vi "FS-Packet over Ethernet Duplex.vi"() -> ()   [LabVIEW 2018]
uses:
  FGV Mode.ctl
  <vilib>/Utility/error.llb/DialogType.ctl
  <instrlib>/niUSRP/niUSRP Write Tx Data (I16).vi
  <instrlib>/niUSRP/niUSRP Fetch Rx Data (I16).vi
panel:
  in  "タブ制御器":enum32{"Settings", "Readback"}(tab)
  in  "device names":refnum<k15>="192.168.1.51"
  in  "number of samples":i64=2000
  in  "IQ rate":dbl=100000.0 format="%#_6p"
  in  "rx carrier frequency":dbl=2000000000.0 format="%#_6p"
  in  "rx gain":dbl format="%#_6f"
  in  "tx gain":dbl format="%#_6f"
  in  "tx carrier frequency":dbl=2000000000.0 format="%#_6p"
  in  "dstaddr":string="192.168.0.112" caption="IQデータ送信先のIPアドレス"
  in  "dsrport":i32=40000 caption="IQデータ送信先のポート番号"
  in  "srcaddr":string="192.168.0.109" caption="IQデータを受信するIPアドレス"
  in  "srcport":i32=40000 caption="IQデータを受信するポート番号"
  in  "UDP socket buffer size (recv)":i32=64000
  in  "rx buff size (max)":i32=500 caption="USRP受信用バッファサイズ"
  in  "USRP送信用バッファサイズ":i32=500
  out "rx buffer (current)":i32
  out "tx buffer (current)":i32
  out "UDP recv bytes":i32
  out "rx IQ rate":dbl=100000.0 format="%#_6p"
  out "rx carrier frequency":dbl=2000000000.0 format="%#_6p"
  out "rx gain 2":dbl format="%#_6f"
  out "tx IQ rate":dbl=100000.0 format="%#_6p"
  out "tx carrier frequency":dbl=2000000000.0 format="%#_6p"
  out "tx gain 2":dbl format="%#_6f"
  out "udp tx loop":errorcluster
  out "udp rx loop":errorcluster
  out "usrp tx loop":errorcluster
  out "usrp rx loop":errorcluster
  in  "停止":bool
  out "UDP Recv timeout":bool
  out "tx buffer full":bool caption="tx buffer full (UDP - USRP)"
  out "rx buffer full":bool caption="rx buffer full (USRP - UDP)"
  out "IQ data":i16[](array[numeric])
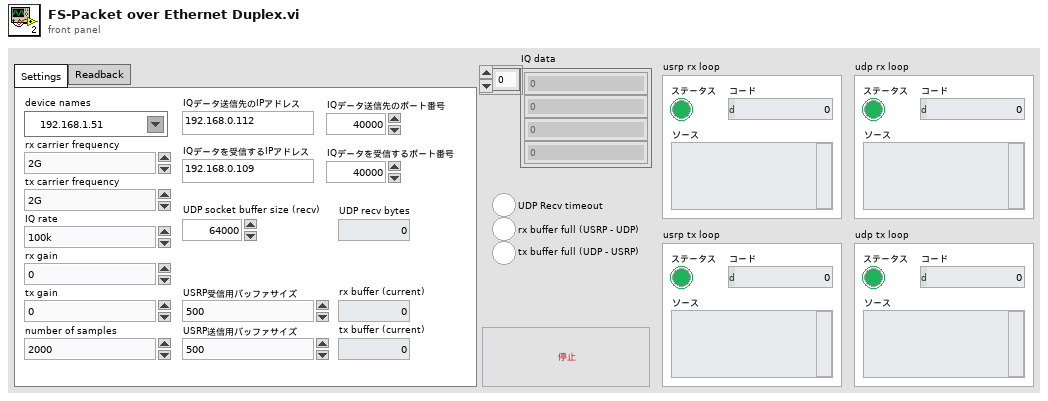
[diagram p1: front panel]
types:
  T1 = typedef "FGV Mode.ctl" = enum16{"None", "Init", "Set", "Get", "Update", "Clear"}
  T2 = typedef "DialogType.ctl" = u16
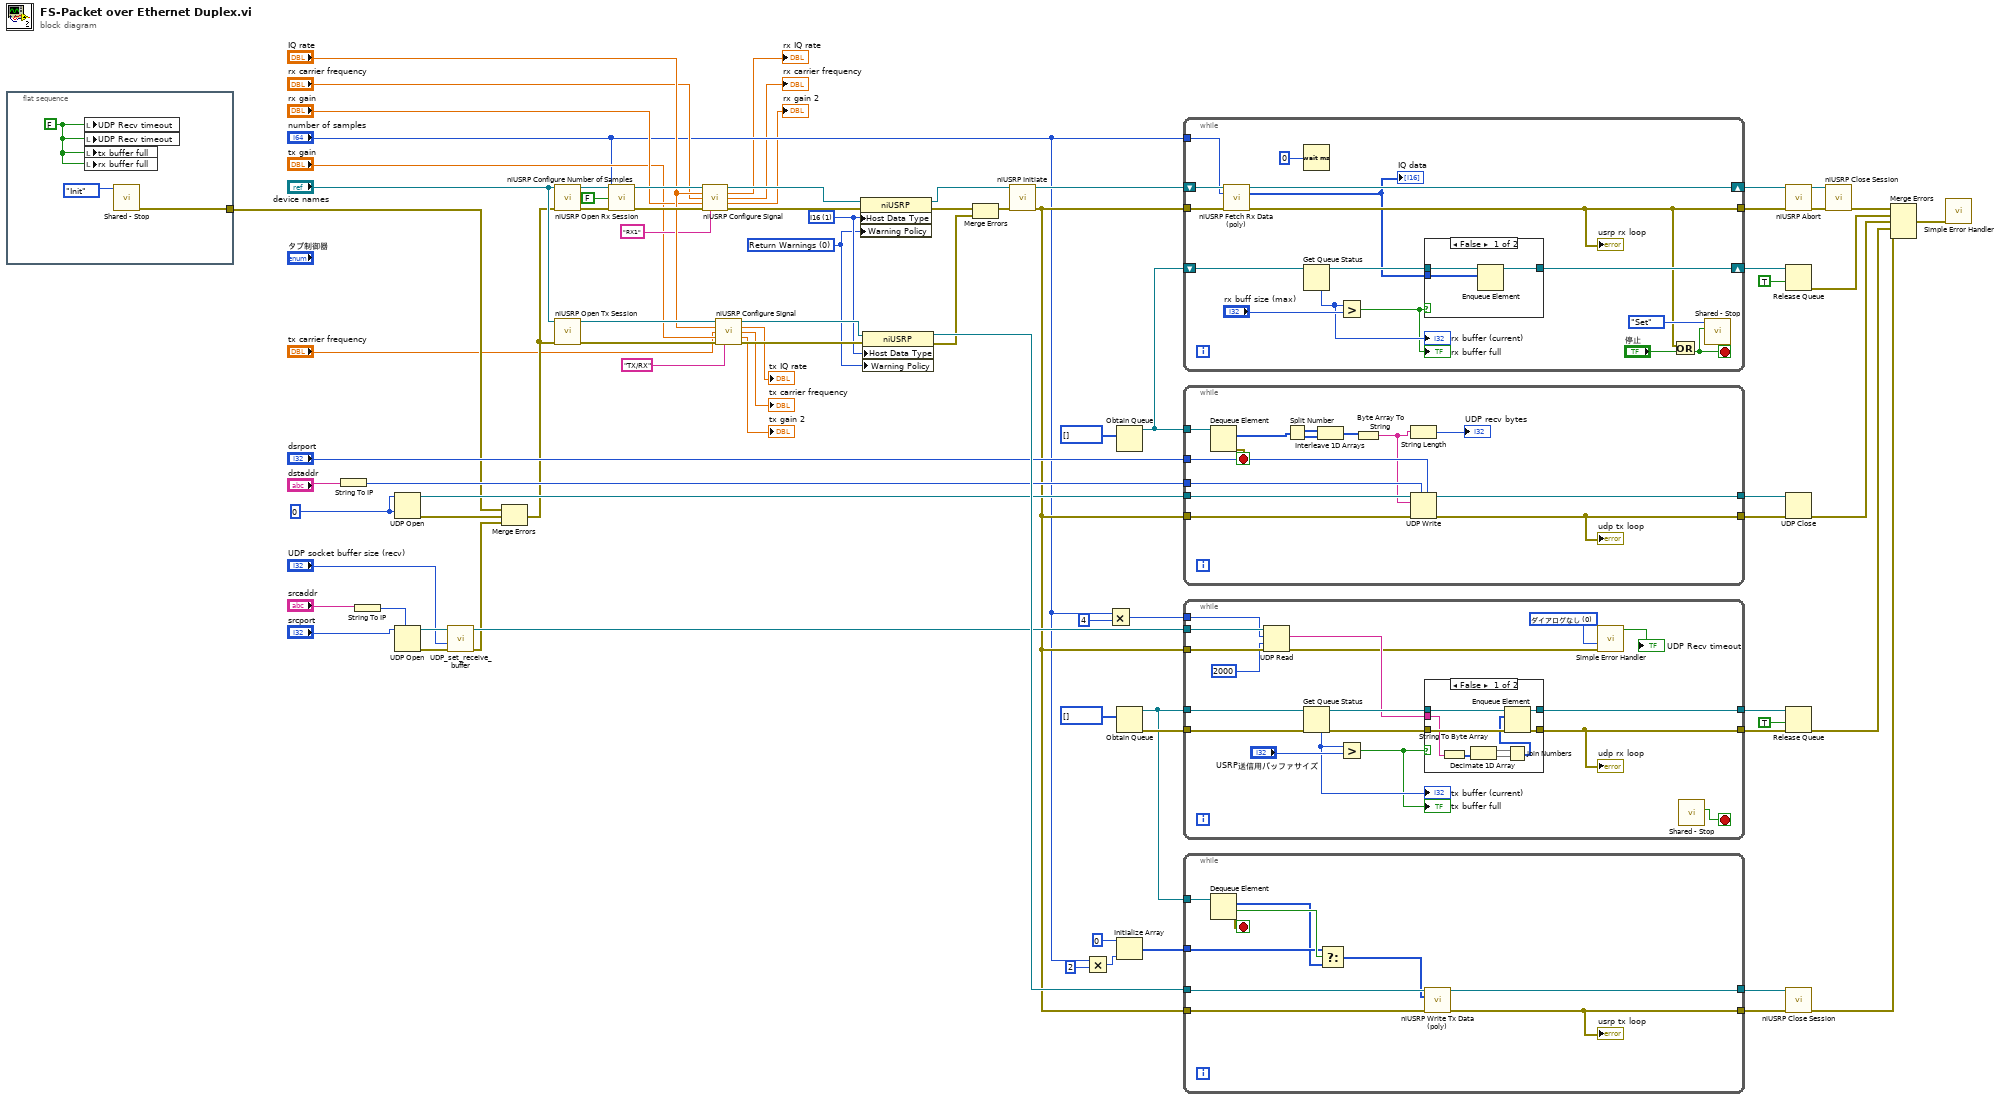
[diagram p0: block diagram]
diagram:
  w47 = u32 0 ("ネットアドレス")
  w18 = 0 items=["Return Warnings", "Return Errors", "Return Success"] ("Configuration:Advanced:Warning Policy")
  w19 = 1 items=["CDB", "I16"] ("Configuration:Advanced:Host Data Type")
  n1 = flat-sequence {
    tunnel: [w82] -> w25
    frame #0 {
      w84 = FALSE ("USRP rx overflow")
      n2 = local write "UDP Recv timeout"(w84) -> ()
      n3 = local write "UDP Recv timeout"(w84) -> ()
      n4 = local write "tx buffer full"(w84) -> ()
      n5 = local write "rx buffer full"(w84) -> ()
      n6 = call "Shared - Stop.vi"("FGV Mode"=FGV_Mode."Init") -> ("error out"=w82:errorcluster)  [unwired: 9 in, 1 out]
    }
  }
  n7 = String To IP(1:"dstaddr") -> (0:w49:u32)
  n8 = String To IP(1:"srcaddr") -> (0:w43:u32)
  n9 = UDP Open(7:w47, 11:w47) -> (port=w52:refnum<k16>, 0:w31:errorcluster)  [unwired: 3 in, 1 out]
  n10 = UDP Open(7:w43, 11:"srcport") -> (port=w36:refnum<k16>, 0:w35:errorcluster)  [unwired: 3 in, 1 out]
  n11 = call "UDP_set_receive_buffer.vi"("error in (no error)"=w35, "Receive Buffer Size"="UDP socket buffer size (recv)", "connection ID"=w36) -> ("error out"=w24:errorcluster, "connection ID out"=w34:refnum<k16>)  [unwired: 6 in]
  n12 = Merge Errors(w25, w31, w24) -> (w23:errorcluster)
  n13 = call <instrlib>:"niUSRP Open Rx Session.vi"("device names"="device names", "error in (no error)"=w23) -> ("session handle out"=w81:refnum<k15>, "error out"=w72:errorcluster)  [unwired: 12 in]
  n14 = call <instrlib>:"niUSRP Open Tx Session.vi"("device names"="device names", "error in (no error)"=w23) -> ("session handle out"=w69:refnum<k15>, "error out"=w68:errorcluster)  [unwired: 12 in]
  n15 = call <instrlib>:"niUSRP Configure Number of Samples.vi"("session handle"=w81, "number of samples is finite"=FALSE, "number of samples"="number of samples", "error in (no error)"=w72) -> ("session handle out"=w80:refnum<k15>, "error out"=w73:errorcluster)  [unwired: 10 in]
  n16 = call <instrlib>:"niUSRP Configure Signal.vi"("session handle"=w80, "IQ rate"="IQ rate", "carrier frequency"="rx carrier frequency", "gain"="rx gain", "error in (no error)"=w73, "active antenna"="RX1") -> ("session handle out"=w79:refnum<k15>, "coerced IQ rate"=→"rx IQ rate":dbl, "coerced carrier frequency"=→"rx carrier frequency":dbl, "coerced gain"=→"rx gain 2":dbl, "error out"=w59:errorcluster)  [unwired: 5 in]
  n17 = call <instrlib>:"niUSRP Configure Signal.vi"("session handle"=w69, "IQ rate"="IQ rate", "carrier frequency"="tx carrier frequency", "gain"="tx gain", "error in (no error)"=w68, "active antenna"="TX/RX") -> ("session handle out"=w58:refnum<k15>, "coerced IQ rate"=→"tx IQ rate":dbl, "coerced carrier frequency"=→"tx carrier frequency":dbl, "coerced gain"=→"tx gain 2":dbl, "error out"=w56:errorcluster)  [unwired: 5 in]
  n18 = property class="niUSRP"(reference=w79, error in=w59, "Host Data Type"=w19, "Warning Policy"=w18) -> (reference out=w60:refnum<k15>, error out=w30:errorcluster)
  n19 = property class="niUSRP"(reference=w58, error in=w56, "Host Data Type"=w19, "Warning Policy"=w18) -> (reference out=w57:refnum<k15>, error out=w21:errorcluster)
  n20 = Merge Errors(w30, w21) -> (w22:errorcluster)
  n21 = call <instrlib>:"niUSRP Initiate.vi"("session handle"=w60, "error in (no error)"=w22) -> ("session handle out"=w78:refnum<k15>, "error out"=w20:errorcluster)  [unwired: 12 in]
  n22 = Multiply(x="number of samples", y=i16 2) -> (x*y=w9:i64)
  n23 = Multiply(x="number of samples", y=4 ("最大サイズ (548)")) -> (x*y=w28:i64)
  n24 = Obtain Queue(element data type=i16[] []) -> (queue out=w53:refnum<queue>)  [unwired: 4 in, 2 out]
  n25 = Obtain Queue(element data type=i16[] []) -> (queue out=w37:refnum<queue>, error out=w41:errorcluster)  [unwired: 4 in, 1 out]
  n26 = Initialize Array(i16 0, w9) -> (w8:i16[])
  n27 = while {
    shift-right: [w99] -> w77
    shift-left: w78 -> [w100]
    tunnel: "number of samples" -> [w96]
    shift-right: [w95] -> w51
    shift-left: w53 -> [w94]
    tunnel: w20 -> [w98]
    tunnel: [w86] -> w74
    stop <- w87 stop-if-true
    n28 = call-poly <instrlib>:"niUSRP Fetch Rx Data (poly).vi"("session handle"=w100, "number of samples"=w96, "error in (no error)"=w98) -> ("session handle out"=w99:refnum<k15>, "data"=w85:i16[], "error out"=w86:errorcluster)  [unwired: 9 in, 1 out]
    "IQ data" <- w85
    "usrp rx loop" <- w86
    n29 = Wait (ms)(milliseconds to wait=u32 0 ("ミリ秒待機時間")) -> ()  [unwired: 1 out]
    n30 = Get Queue Status(queue=w94) -> (queue out=w93:refnum<queue>, # elements in queue=w90:i32)  [unwired: 2 in, 6 out]
    "rx buffer (current)" <- w90
    n31 = Greater?(x=w90, y="rx buff size (max)") -> (0:w89:bool)
    "rx buffer full" <- w89
    n32 = case shown="FALSE" w89 {
      tunnel: [w103 w104] -> w95
      tunnel: w93 -> [w102 w104]
      tunnel: w85 -> [w101 _]
      frame False {
        n33 = Enqueue Element(queue=w102, element=w101) -> (queue out=w103:refnum<queue>)  [unwired: 2 in, 2 out]
      }
      frame True {
      }
    }
    n34 = Or(x=w86, y="停止") -> (x .or. y?=w87:bool)
    n35 = call "Shared - Stop.vi"("Stop in"=w87, "FGV Mode"=FGV_Mode."Set") -> ()  [unwired: 8 in, 2 out]
  }
  n36 = while {
    tunnel: w53 -> [w118]
    tunnel: w52 -> [w116]
    tunnel: w49 -> [w111]
    tunnel: "dsrport" -> [w110]
    tunnel: w20 -> [w109]
    tunnel: [w108] -> w46
    tunnel: [w105] -> w45
    stop <- w117 stop-if-true
    n37 = Dequeue Element(queue=w118) -> (element=w115:i16[], error out=w117:errorcluster)  [unwired: 2 in, 2 out]
    n38 = Split Number(x=w115) -> (hi(x)=w114:u8[], lo(x)=w113:u8[])
    n39 = Interleave 1D Arrays(w114, w113) -> (w112:u8[])
    n40 = Byte Array To String(unsigned byte array=w112) -> (string=w107:string)
    n41 = String Length(string=w107) -> (length=→"UDP recv bytes":i32)
    n42 = UDP Write(address=w111, port or service name=w110, connection ID=w116, data in=w107, 8:w109) -> (error out=w105:errorcluster, 3:w108:refnum<k16>)  [unwired: 1 in]
    "udp tx loop" <- w105
  }
  n43 = while {
    tunnel: w34 -> [w136]
    tunnel: w20 -> [w135]
    tunnel: w37 -> [w133]
    tunnel: w41 -> [w132]
    tunnel: [w129] -> w39
    tunnel: [w119] -> w38
    tunnel: w28 -> [w125]
    stop <- w127 stop-if-true
    w122 = T2 0 items=["ダイアログなし", "OKメッセージ", "継続か停止メッセージ", "OKメッセージ+警告", "継続/停止+警告"] ("type of dialog (OK msg:1)")
    n44 = UDP Read(connection ID=w136, max size (548)=w125, timeout ms (25000)=2000 ("タイムアウト (ms) (25000)"), 8:w135) -> (data out=w131:string, error out=w124:errorcluster)  [unwired: 3 out]
    n45 = Get Queue Status(queue=w133, error in (no error)=w132) -> (queue out=w134:refnum<queue>, error out=w128:errorcluster, # elements in queue=w121:i32)  [unwired: 1 in, 5 out]
    "tx buffer (current)" <- w121
    n46 = Greater?(x=w121, y="USRP送信用バッファサイズ") -> (0:w120:bool)
    "tx buffer full" <- w120
    n47 = case shown="FALSE" w120 {
      tunnel: [w145 w147] -> w129
      tunnel: w134 -> [w144 w147]
      tunnel: w131 -> [w138 _]
      tunnel: w128 -> [w143 w146]
      tunnel: [w142 w146] -> w119
      frame False {
        n48 = String To Byte Array(string=w138) -> (unsigned byte array=w139:u8[])
        n49 = Decimate 1D Array(w139) -> (w140:u8[], w141:u8[])
        n50 = Join Numbers(hi=w140, lo=w141) -> ((hi.lo)=w137:u16[])
        n51 = Enqueue Element(queue=w144, element=w137, error in (no error)=w143) -> (queue out=w145:refnum<queue>, error out=w142:errorcluster)  [unwired: 1 in, 1 out]
      }
      frame True {
      }
    }
    "udp rx loop" <- w119
    n52 = call <vilib>:"Simple Error Handler.vi"("type of dialog (OK msg:1)"=w122, "error in (no error)"=w124) -> ("error?"=→"UDP Recv timeout":bool)  [unwired: 3 in, 4 out]
    n53 = call "Shared - Stop.vi"() -> ("Stop out"=w127:bool)  [unwired: 10 in, 1 out]
  }
  n54 = while {
    tunnel: w57 -> [w157]
    tunnel: [w156] -> w63
    tunnel: [w153] -> w62
    tunnel: w37 -> [w155]
    tunnel: w20 -> [w152]
    tunnel: w8 -> [w150]
    stop <- w154 stop-if-true
    n55 = Dequeue Element(queue=w155) -> (element=w148:i16[], timed out?=w151:bool, error out=w154:errorcluster)  [unwired: 2 in, 1 out]
    n56 = Select(t=w150, s=w151, f=w148) -> (s? t:f=w149:i16[])
    n57 = call-poly <instrlib>:"niUSRP Write Tx Data (poly).vi"("session handle"=w157, "data"=w149, "error in (no error)"=w152) -> ("session handle out"=w156:refnum<k15>, "error out"=w153:errorcluster)  [unwired: 11 in]
    "usrp tx loop" <- w153
  }
  n58 = call <instrlib>:"niUSRP Abort.vi"("session handle"=w77, "error in (no error)"=w74) -> ("session handle out"=w76:refnum<k15>, "error out"=w75:errorcluster)  [unwired: 12 in]
  n59 = Release Queue(queue=w51, force destroy? (F)=TRUE ("破棄を強制? (F)")) -> (error out=w16:errorcluster)  [unwired: 1 in, 2 out]
  n60 = UDP Close(connection ID=w46, 8:w45) -> (error out=w15:errorcluster)  [unwired: 1 out]
  n61 = Release Queue(queue=w39, force destroy? (F)=TRUE ("破棄を強制? (F)"), error in (no error)=w38) -> (error out=w14:errorcluster)  [unwired: 2 out]
  n62 = call <instrlib>:"niUSRP Close Session.vi"("session handle"=w63, "error in (no error)"=w62) -> ("error out"=w13:errorcluster)  [unwired: 13 in]
  n63 = call <instrlib>:"niUSRP Close Session.vi"("session handle"=w76, "error in (no error)"=w75) -> ("error out"=w33:errorcluster)  [unwired: 13 in]
  n64 = Merge Errors(w33, w16, w15, w14, w13) -> (w17:errorcluster)
  n65 = call <vilib>:"Simple Error Handler.vi"("error in (no error)"=w17) -> ()  [unwired: 4 in, 5 out]
